vi "Generate Default Project Name and Path.vi"(11 "DNL_MetaDataObj in":refnum<class "MetaDataObj.lvclass">) -> (1 "Project Root":path caption="项目根目录", 2 "Project Name":string caption="项目名称", 3 "DNL_MetaDataObj out":refnum<class "MetaDataObj.lvclass">)   [LabVIEW 2016]
uses:
  <resource>/dialog/NewProjectWizard/MetaDataObj/MetaDataObj.lvclass
  <resource>/dialog/NewProjectWizard/MetaDataObj/MetaDataObj.lvclass/MetaDataObj.ctl
  <resource>/dialog/NewProjectWizard/MetaDataObj/Accessors/Read Project Root.vi
  <resource>/dialog/NewProjectWizard/MetaDataObj/Accessors/Write Project Root.vi
  <resource>/dialog/NewProjectWizard/MetaDataObj/Accessors/Write Project Name.vi
panel:
  in  "Untitled Project Name":string="未命名项目%d" caption="未命名项目名称"
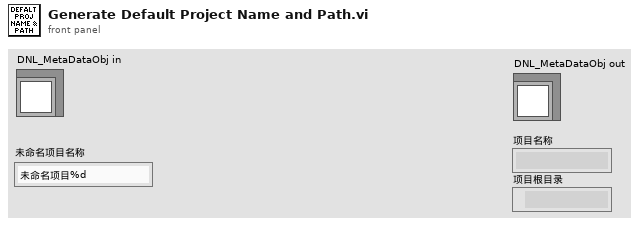
[diagram p1: front panel]
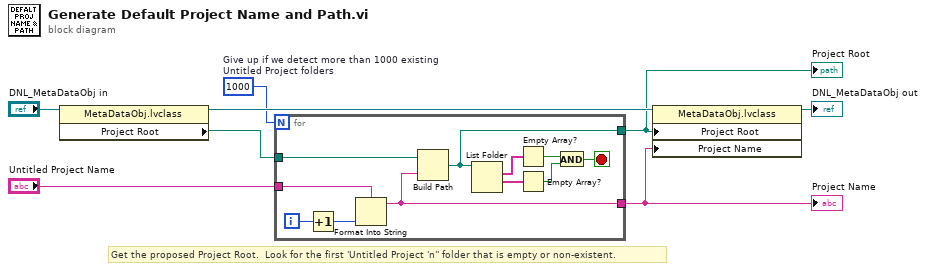
[diagram p0: block diagram]
diagram:
  w2 = 1000  # Give up if we detect more than 1000 existing Untitled Project folders
  # "Get the proposed Project Root.  Look for the first 'Untitled Project 'n'' folder that is empty or non-existent."
  n1 = property class="MetaDataObj.lvclass"(reference="DNL_MetaDataObj in") -> (reference out=w7:refnum<class "MetaDataObj.lvclass">, "Project Root"=w1:path)  [unwired: 1 in, 1 out]
  n2 = for {
    N: w2 -> [_]
    tunnel: w1 -> [w19]
    tunnel: "Untitled Project Name" -> [w18]
    tunnel: [w11] -> w4
    tunnel: [w10] -> w3
    i -> [w17]
    stop <- w9 stop-if-true
    n3 = Increment(x=w17) -> (x+1=w16:i32)
    n4 = Format Into String(format string=w18, w16) -> (resulting string=w11:string)  [unwired: 2 in, 1 out]
    n5 = Build Path(base path=w19, name or relative path=w11) -> (appended path=w10:path)
    n6 = List Folder(path=w10) -> (filenames=w15:string[], folder names=w14:string[])  [unwired: 3 in, 2 out]
    n7 = Empty Array?(array=w15) -> (empty?=w13:bool)
    n8 = Empty Array?(array=w14) -> (empty?=w12:bool)
    n9 = And(x=w13, y=w12) -> (x .and. y?=w9:bool)
  }
  "Project Name" <- w4
  "Project Root" <- w3
  n10 = property class="MetaDataObj.lvclass"(reference=w7, "Project Root"=w3, "Project Name"=w4) -> (reference out=→"DNL_MetaDataObj out":refnum<class "MetaDataObj.lvclass">)  [unwired: 1 in, 1 out]
